vi "Burner.vi"() -> ()   [LabVIEW 2019]
panel:
  out "length":i32
  in  "?":bool
  in  "Select the serial port with wio from the list":u16(ring) items=["/dev/cu.Bluetooth-Incoming-Port", "/dev/cu.LEGOHubMilan-SerialPort", "/dev/cu.usbmodem14201"]
  out "OUTPUT CONSOLE":string
  out "ERROR":string
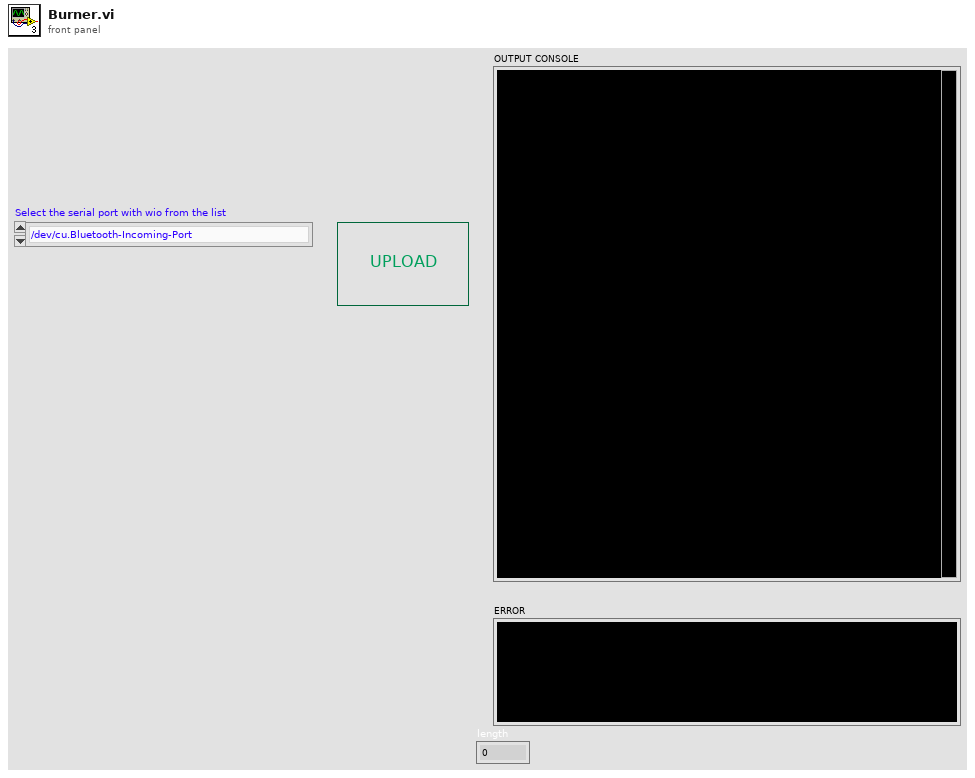
[diagram p1: front panel]
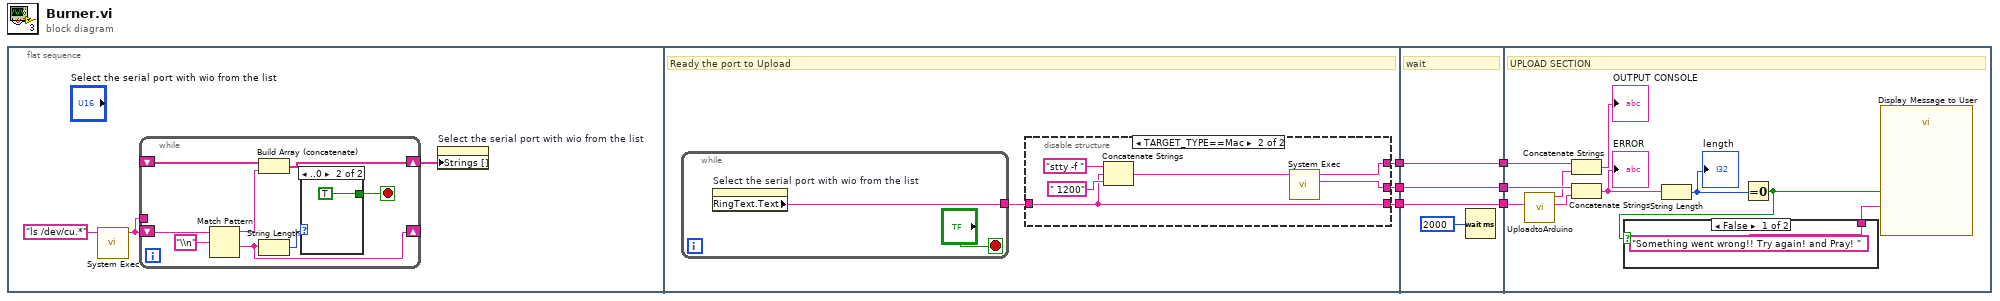
[diagram p0: block diagram]
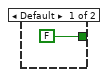
[diagram p2: hidden frame]
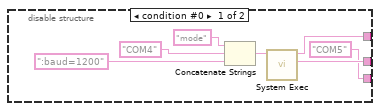
[diagram p3: hidden frame]
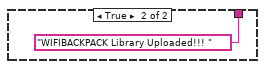
[diagram p4: hidden frame]
diagram:
  n1 = flat-sequence {
    tunnel: [w21] -> w6
    tunnel: [w22] -> w3
    tunnel: [w23] -> w2
    tunnel: w6 -> [w41]
    tunnel: [w41] -> w5
    tunnel: [w40] -> w4
    tunnel: w3 -> [w40]
    tunnel: w2 -> [w39]
    tunnel: [w39] -> w1
    tunnel: w5 -> [w47]
    tunnel: w4 -> [w52]
    tunnel: w1 -> [w50]
    frame #0 {
      n2 = call <vilib>:"System Exec.vi"("command line"="ls /dev/cu.*") -> ("standard output"=w7:string)  [unwired: 7 in, 3 out]
      n3 = while {
        tunnel: w7 -> [_]
        shift-right: [w14] -> w8
        shift-left: _ -> [w15]
        shift-right: [w10] -> _
        shift-left: w7 -> [w11]
        stop <- w12 stop-if-true
        n4 = Match Pattern(string=w11, regular expression="\\n") -> (before substring=w16:string, after substring=w10:string)  [unwired: 1 in, 2 out]
        n5 = Build Array (concatenate)(w15, w16) -> (w14:string[])
        n6 = String Length(string=w10) -> (length=w13:i32)
        n7 = case shown="..0" w13 {
          tunnel: [FALSE TRUE] -> w12
          frame Default {
          }
          frame ..0 {
          }
        }
      }
      n8 = property on="Select the serial port with wio from the list" class="Ring (strict)"("Strings []"=w8) -> ()  [unwired: 2 in, 2 out]
    }
    frame #1 {
      # "Ready the port to Upload"
      n9 = while {
        tunnel: [w24] -> w20
        stop <- "?" stop-if-true
        n10 = property on="Select the serial port with wio from the list" class="Ring (strict)"() -> ("RingText.Text"=w24:string)  [unwired: 2 in, 2 out]
      }
      n11 = disable-structure shown="TARGET_TYPE==Mac" {
        disable-tunnel: [w28 w35] -> w23
        disable-tunnel: [w27 w34] -> w22
        disable-tunnel: ["COM5" ("string") w33] -> w21
        disable-tunnel: w20 -> [_ w33]
        frame condition #0 {
          n12 = Concatenate Strings("mode" ("string"), "COM4" ("string"), ":baud=1200" ("string")) -> (w32:string)
          n13 = call <vilib>:"System Exec.vi"("command line"=w32) -> ("standard error"=w27:string, "standard output"=w28:string)  [unwired: 7 in, 2 out]
        }
        frame condition #1 (active) {
          n14 = Concatenate Strings("stty -f " ("string"), w33, " 1200" ("string")) -> (w38:string)
          n15 = call <vilib>:"System Exec.vi"("command line"=w38) -> ("standard error"=w34:string, "standard output"=w35:string)  [unwired: 7 in, 2 out]
        }
      }
    }
    frame #2 {
      # "wait"
      n16 = Wait (ms)(milliseconds to wait=u32 2000) -> ()  [unwired: 1 out]
    }
    frame #3 {
      # "UPLOAD SECTION"
      n17 = call "UploadtoArduino.vi"("serial port"=w47) -> ("standard error"=w51:string, "standard output"=w49:string)  [unwired: 9 in]
      n18 = Concatenate Strings(w50, w49) -> (→"OUTPUT CONSOLE":string)
      n19 = Concatenate Strings(w52, w51) -> (w46:string)
      "ERROR" <- w46
      n20 = String Length(string=w46) -> (length=w45:i32)
      "length" <- w45
      n21 = Equal To 0?(x=w45) -> (x = 0?=w43:bool)
      n22 = case shown="False" w43 {
        tunnel: ["Something went wrong!! Try again! and Pray! " "WIFIBACKPACK Library Uploaded!!! "] -> w44
        frame False {
        }
        frame True {
        }
      }
      n23 = call "Display Message to User"("Enable"=w43, "Message"=w44) -> ()  [unwired: 8 in, 2 out]
    }
  }
